vi "encoder reset.vi"() -> ()   [LabVIEW 2016]
panel:
  out "3NC0D3R R3537":bool
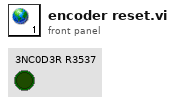
[diagram p1: front panel]
diagram:
